vi "CheckRefs.vi"(9 "All Refs Array Refnum":refnum<vi>, 10 "Array of label refnums":refnum<vi>[](array[refnum]), 11 "Path to refs":path=path "Z:/Programmes en Developpement/octo-labview/Turning Box PI Near Field/Moteurs PI/PI Refs") -> (0 "error out":errorcluster)   [LabVIEW 2014]
panel:
  in  "RefLabels 4":string(combo)
  in  "RefLabels 3":string(combo)
  in  "RefLabels 2":string(combo)
  in  "RefLabels 1":string(combo)
  in  "All refs":dbl[][](array[numeric]) format="%.6f"
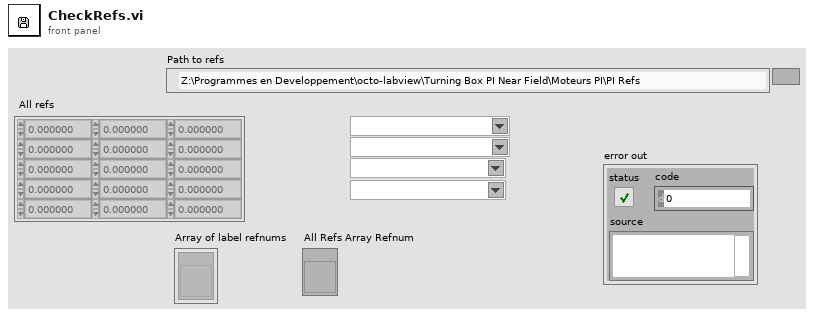
[diagram p1: front panel]
types:
  T1 = enum16{"open", "replace", "create", "open or create", "replace or create", "replace or create with confirmation"}
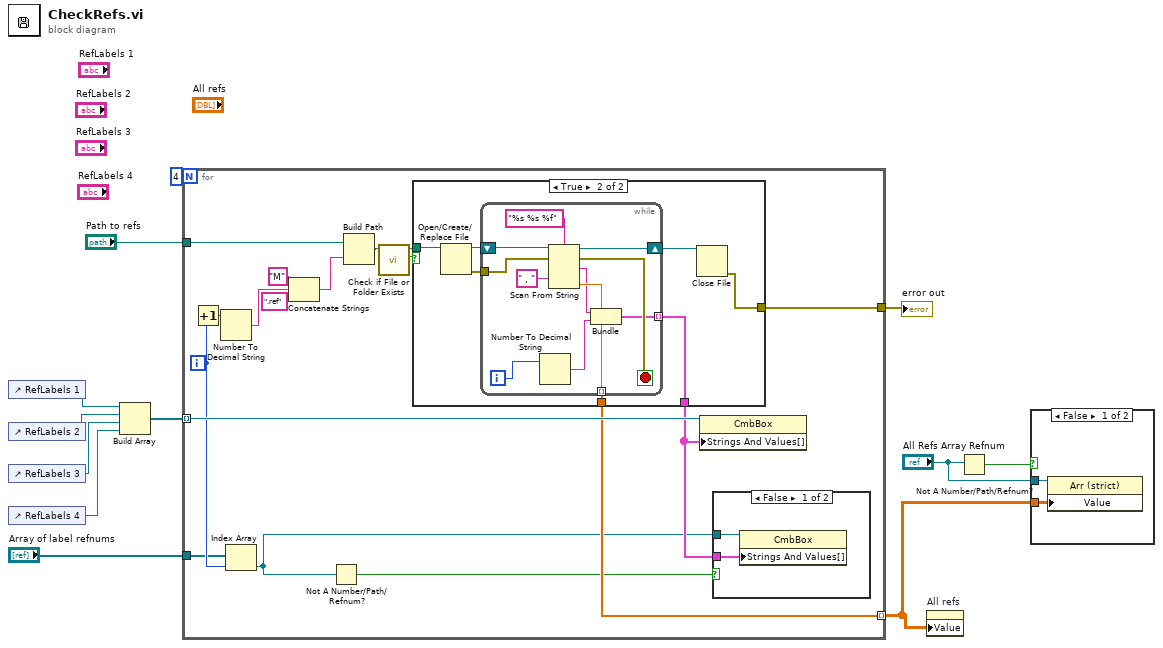
[diagram p0: block diagram]
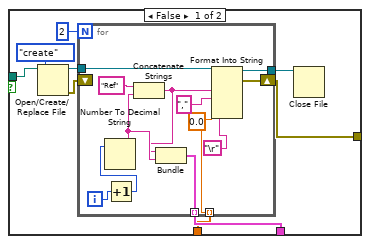
[diagram p4: hidden frame]
diagram:
  n1 = control-ref of="RefLabels 1"() -> (w10:refnum<vi>)
  n2 = control-ref of="RefLabels 2"() -> (w9:refnum<vi>)
  n3 = control-ref of="RefLabels 3"() -> (w8:refnum<vi>)
  n4 = control-ref of="RefLabels 4"() -> (w7:refnum<vi>)
  n5 = Build Array(w10, w9, w8, w7) -> (w6:refnum<vi>[])
  n6 = for {
    N: 4 -> [_]
    tunnel: "Path to refs" -> [w29]
    tunnel: w6 -> [w20] mode=indexing
    tunnel: [w19] -> w3 mode=indexing
    tunnel: [w18] -> w5
    tunnel: "Array of label refnums" -> [w14]
    i -> [w15]
    n7 = Increment(x=w15) -> (x+1=w26:i32)
    n8 = Number To Decimal String(number=w26) -> (decimal integer string=w25:string)  [unwired: 1 in]
    n9 = Index Array(array=w14, index=w15) -> (element=w13:refnum<vi>)
    n10 = Concatenate Strings("M", w25, ".ref") -> (w24:string)
    n11 = Not A Number/Path/Refnum?(number/path/refnum=w13) -> (NaN/Path/Refnum?=w16:bool)
    n12 = Build Path(base path=w29, name or relative path=w24) -> (appended path=w23:path)
    n13 = call <vilib>:"Check if File or Folder Exists.vi"("path"=w23) -> ("file or folder exists?"=w22:bool, "dup path"=w21:path)  [unwired: 8 in, 1 out]
    n14 = case shown="True" w22 {
      tunnel: w21 -> [w37 w59]
      tunnel: [w34 w53] -> w17
      tunnel: [w33 w55] -> w19
      tunnel: [w32 w54] -> w18
      frame False {
        n15 = Open/Create/Replace File(file path (use dialog)=w37, operation (0:open)=T1."create") -> (refnum out=w40:refnum<file>, error out=w39:errorcluster)  [unwired: 4 in, 1 out]
        n16 = for {
          N: 2 -> [_]
          tunnel: w40 -> [w52]
          tunnel: [w49] -> w35
          tunnel: [w42] -> w34 mode=indexing
          tunnel: [w47] -> w33 mode=indexing
          shift-right: [w45] -> w32
          shift-left: w39 -> [_]
          i -> [w50]
          w47 = 0.0
          n17 = Increment(x=w50) -> (x+1=w48:i32)
          n18 = Number To Decimal String(number=w48) -> (decimal integer string=w44:string)  [unwired: 1 in]
          n19 = Concatenate Strings("Ref", w44) -> (w43:string)
          n20 = Bundle(w43, w44) -> (w42:cluster{string, string})  [unwired: 1 in]
          n21 = Format Into String(initial string=w52, w43, ",", w47, "\r") -> (resulting string=w49:refnum<file>, error out=w45:errorcluster)  [unwired: 2 in]
        }
        n22 = Close File(refnum=w35) -> ()  [unwired: 1 in, 2 out]
      }
      frame True {
        n23 = Open/Create/Replace File(file path (use dialog)=w59) -> (refnum out=w58:refnum<file>, error out=w57:errorcluster)  [unwired: 5 in, 1 out]
        n24 = while {
          tunnel: w57 -> [w67]
          tunnel: [w66] -> w55 mode=indexing
          tunnel: [w62] -> w53 mode=indexing
          shift-right: [w69] -> w56
          shift-left: w58 -> [w70]
          i -> [w65]
          stop <- w68 stop-if-true
          n25 = Number To Decimal String(number=w65) -> (decimal integer string=w63:string)  [unwired: 1 in]
          n26 = Scan From String("%s %s %f" ("format string"), w70, w67, default 2=" , ") -> (w69:refnum<file>, w68:errorcluster, output 1=w64:string, output 3=w66:dbl)  [unwired: 3 in]
          n27 = Bundle(w64, w63) -> (w62:cluster{string, string})  [unwired: 1 in]
        }
        n28 = Close File(refnum=w56) -> (error out=w54:errorcluster)  [unwired: 1 in, 1 out]
      }
    }
    n29 = property class="CmbBox"(reference=w20, "Strings And Values[]"=w17) -> ()  [unwired: 1 in, 2 out]
    n30 = case shown="False" w16 {
      tunnel: w17 -> [w31 _]
      tunnel: w13 -> [w30 _]
      frame False {
        n31 = property class="CmbBox"(reference=w30, "Strings And Values[]"=w31) -> ()  [unwired: 1 in, 2 out]
      }
      frame True {
      }
    }
  }
  "error out" <- w5
  n32 = property on="All refs" class="Arr (strict)"("Value"=w3) -> ()  [unwired: 2 in, 2 out]
  n33 = Not A Number/Path/Refnum?(number/path/refnum="All Refs Array Refnum") -> (NaN/Path/Refnum?=w4:bool)
  n34 = case shown="False" w4 {
    tunnel: w3 -> [w72 _]
    tunnel: "All Refs Array Refnum" -> [w71 _]
    frame False {
      n35 = property class="Arr (strict)"(reference=w71, "Value"=w72) -> ()  [unwired: 1 in, 2 out]
    }
    frame True {
    }
  }
